vi "Get Relay Indexes w Positive Count.vi"(8 "error in (no error)":errorcluster, 9 "Relay Indexes":i32[](array[numeric]), 10 "Relay Counts":i32[](array[numeric])) -> (0 "error out":errorcluster, 1 "Positive Relay Count Array":i32[](array[numeric]))   [LabVIEW 2016, in "SLSC Switch.lvlib" / "SLSC Switch.lvclass"]
uses:
  SLSC Switch.lvclass
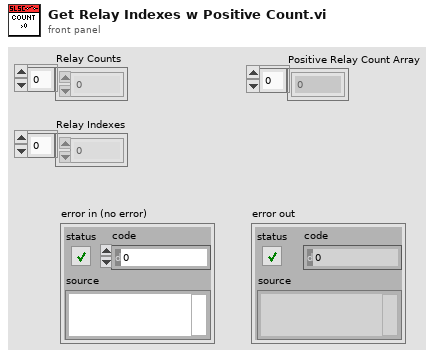
[diagram p1: front panel]
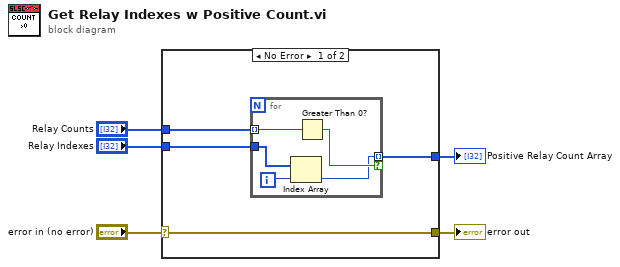
[diagram p0: block diagram]
diagram:
  n1 = case shown="No Error" "error in (no error)" {
    selector: "error in (no error)" -> [w6 w15]
    tunnel: [w9 _] -> w5
    tunnel: "Relay Counts" -> [w8 _]
    tunnel: "Relay Indexes" -> [w7 _]
    tunnel: [w6 w15] -> w1
    frame No Error {
      n2 = for {
        tunnel: w8 -> [w14] mode=indexing
        tunnel: [w12] -> w9 mode=indexing if=w13
        tunnel: w7 -> [w11]
        i -> [w10]
        n3 = Index Array(array=w11, index=w10) -> (element=w12:i32)
        n4 = Greater Than 0?(x=w14) -> (x > 0?=w13:bool)
      }
    }
    frame Error {
    }
  }
  "Positive Relay Count Array" <- w5
  "error out" <- w1
